vi "18.2.1 Color Spectrum.vi"() -> ()   [LabVIEW 2017]
doc: "This example illustrates the use of the horizontal clamp tool. You can draw a region of inspection that contains at least two edges in the image. The VI measures the distance between the first and last edges."
uses:
  <vilib>/vision/NI_Vision_Development_Module.lvlib
panel:
  out "Waveform Chart":dbl[](graph)
  out "Color Spectrum":dbl[](array[numeric]) format="%.2f"
  out "Image":T1(plugin-control)
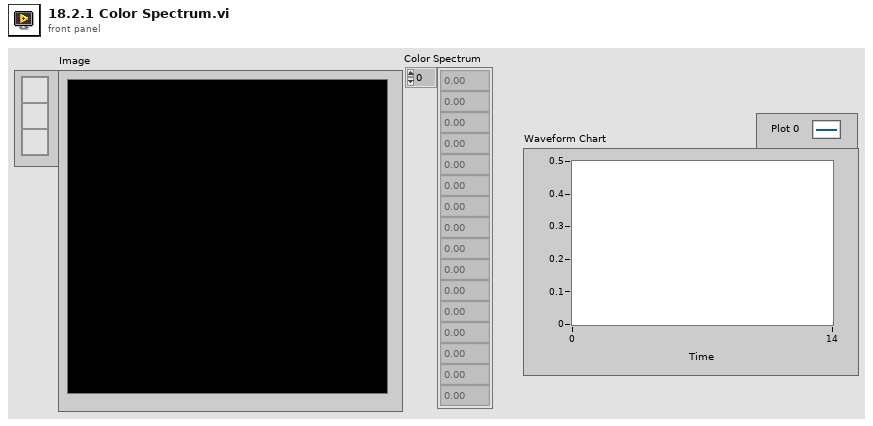
[diagram p1: front panel]
types:
  T1 = typedef "IMAQ Image.ctl" = refnum<image>
  T2 = typedef "Image Type" = u32
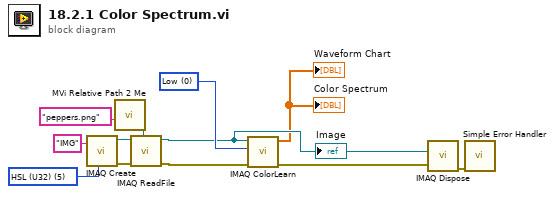
[diagram p0: block diagram]
diagram:
  w2 = T2 5 items=["Grayscale (U8)", "Grayscale (I16)", "Grayscale (SGL)", "Complex (CSG)", "RGB (U32)", "HSL (U32)", "RGB (U64)", "Grayscale (U16)"] ("Image Type")
  w5 = u32 0 items=["Low", "Medium", "High"] ("Color Sensitivity")
  n1 = call "IMAQ Create"("Image Name"="IMG", "Image Type"=w2) -> ("New Image"=w11:T1, "error out"=w10:errorcluster)  [unwired: 3 in]
  n2 = call "MVi Relative Path 2 Me.vi"("Relative Path"="peppers.png" ("name or relative path")) -> ("Appended Dir"=w7:path)  [unwired: 5 in, 1 out]
  n3 = call "IMAQ ReadFile"("File Path"=w7, "error in (no error)"=w10, "Image"=w11) -> ("error out"=w6:errorcluster, "Image Out"=w3:T1)  [unwired: 4 in, 3 out]
  "Image" <- w3
  n4 = call "IMAQ ColorLearn"("Image"=w3, "Color Sensitivity"=w5, "error in (no error)"=w6) -> ("Color Spectrum"=→"Color Spectrum" →"Waveform Chart":dbl[], "error out"=w4:errorcluster)  [unwired: 5 in]
  n5 = call "IMAQ Dispose"("Image"=w3, "error in (no error)"=w4) -> ("error out"=w12:errorcluster)  [unwired: 4 in]
  n6 = call <vilib>:"Simple Error Handler.vi"("error in (no error)"=w12) -> ()  [unwired: 4 in, 5 out]
